vi "test_gmap-dot-net.vi"() -> ()   [LabVIEW 2019]
uses:
  C:/Users/WeGo/Documents/GitHub/Ycar/LabVIEW/Gmap/dll/GMap.NET.WindowsForms.dll
  dll/GMap.NET.WindowsForms.dll
  C:/Users/WeGo/Documents/GitHub/Ycar/LabVIEW/Gmap/dll/GMap.NET.Core.dll
  dll/GMap.NET.Core.dll
  System.Drawing
panel:
  in  "탭 컨트롤":enum32{"페이지 1", "페이지 2"}(tab)
  in  "SetMapProvider":u16(ring)=12 items=["None", "OpenStreetMap", "OpenStreet4UMap", "OpenCycleMap", "OpenCycleLandscapeMap", "OpenCycleTransportMap", "OpenStreetMapQuest", "OpenStreetMapQuestSattelite", "OpenStreetMapQuestHybrid", "OpenSeaMapHybrid", "WikiMapiaMap", "BingMap", "BingSatelliteMap", "BingHybridMap", "YahooMap", "YahooSatelliteMap", "YahooHybridMap", "GoogleMap", "GoogleSatelliteMap", "GoogleHybridMap", "GoogleTerrainMap", "GoogleChinaMap", "GoogleChinaSatelliteMap", "GoogleChinaHybridMap", "GoogleChinaTerrainMap", "GoogleKoreaMap", "GoogleKoreaSatelliteMap", "GoogleKoreaHybridMap", "NearMap", "NearSatelliteMap", "NearHybridMap", "OviMap", "OviSatelliteMap", "OviHybridMap", "OviTerrainMap", "YandexMap", "YandexSatelliteMap", "YandexHybridMap", "LithuaniaMap", "Lithuania 2.5d Map", "LithuaniaOrtoFotoMap", "LithuaniaOrtoFotoMapOld", "LithuaniaHybridMap", "LithuaniaHybridMapOld", "LithuaniaTOP50", "LatviaMap", "MapBender, WMS demo", "TurkeyMap", "CloudMade, Demo", "SpainMap", "CzechMap", "CzechSatelliteMap", "CzechHybridMap", "CzechTuristMap", "CzechHistoryMap", "ArcGIS_Imagery_World_2D_Map", "ArcGIS_ShadedRelief_World_2D_Map", "ArcGIS_StreetMap_World_2D_Map", "ArcGIS_Topo_US_2D_Map", "ArcGIS_World_Physical_Map", "ArcGIS_World_Shaded_Relief_Map", "ArcGIS_World_Street_Map", "ArcGIS_World_Terrain_Base_Map", "ArcGIS_World_Topo_Map", "ArcGIS_DarbAE_Q2_2011_NAVTQ_Eng_V5_MapProvider"]
  in  "GMapControl":refnum<k24>(container)
  in  "정지":bool
  in  "delay":u32=222
  in  "scale":dbl(slide) scale=0.0..20.0
  in  "keys":string
  out "SetPositionByKeywords":i32(ring)=200 items=["G_GEO_SUCCESS"=200, "G_GEO_BAD_REQUEST"=400, "G_GEO_SERVER_ERROR"=500, "G_GEO_MISSING_ADDRESS, G_GEO_MISSING_QUERY"=601, "G_GEO_UNKNOWN_ADDRESS"=602, "G_GEO_UNAVAILABLE_ADDRESS"=603, "G_GEO_UNKNOWN_DIRECTIONS"=604, "G_GEO_BAD_KEY"=610, "G_GEO_TOO_MANY_QUERIES"=620, "ExceptionInCode"=621, "Unknow"=-1]
  in  "MouseLat":dbl format="%.13f"
  in  "MouseLog":dbl format="%.13f"
  in  "MouseLat_DbClk":dbl format="%.13f"
  in  "MouseLog_DbClk":dbl format="%.13f"
  in  "PinDropLat_DblClk":dbl format="%.13f"
  in  "PinDropLon_DblClk":dbl format="%.13f"
  in  "dt":u32=150
  out "error out":errorcluster
  out "Contains":bool
  out "배열":cluster{string, string}[](array[cluster])
  out "Data":u8[](array[numeric])
  out "숫자형":i32
  out "Count":i32
  out "배열 2":T1(array[cluster])
  out "n":i32
  in  "keys 2":string
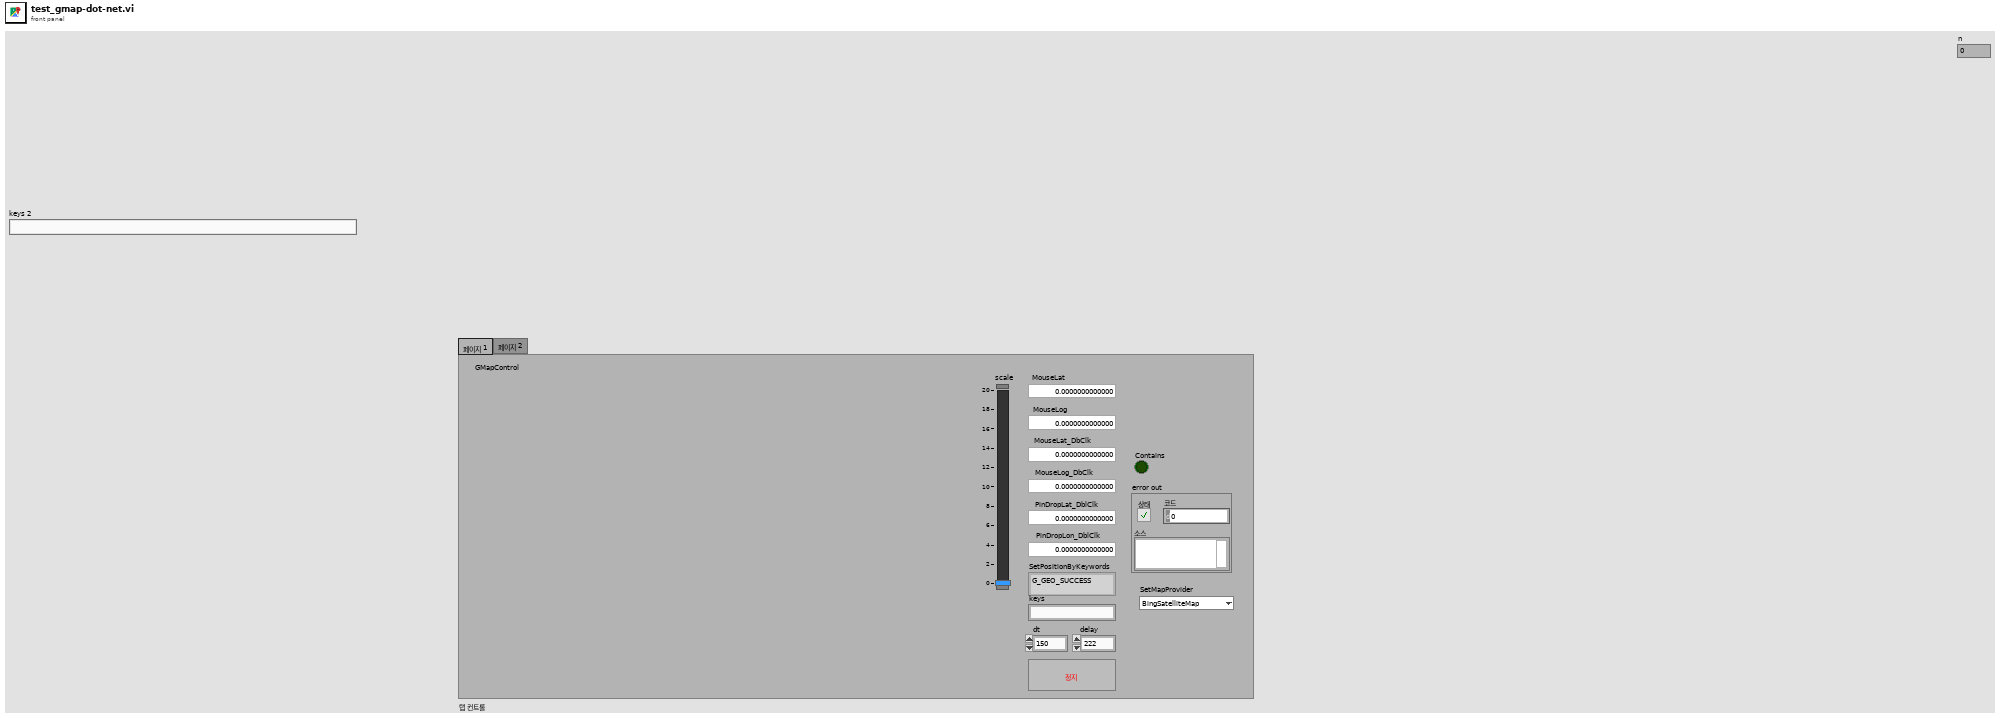
[diagram p1: front panel]
types:
  T1 = cluster{"index":i32, "dotnetrefs":refnum<k24>, "Name":string}[]
  T2 = typedef "mapinfo.ctl" = cluster{"GmapDotNet":refnum<k24>, "mapprovider_info":cluster{"index":i32, "dotnetrefs":refnum<k24>, "Name":string}[]}
  T3 = cluster{"index":i32, "dotnetrefs":refnum<k24>, "Name":string}
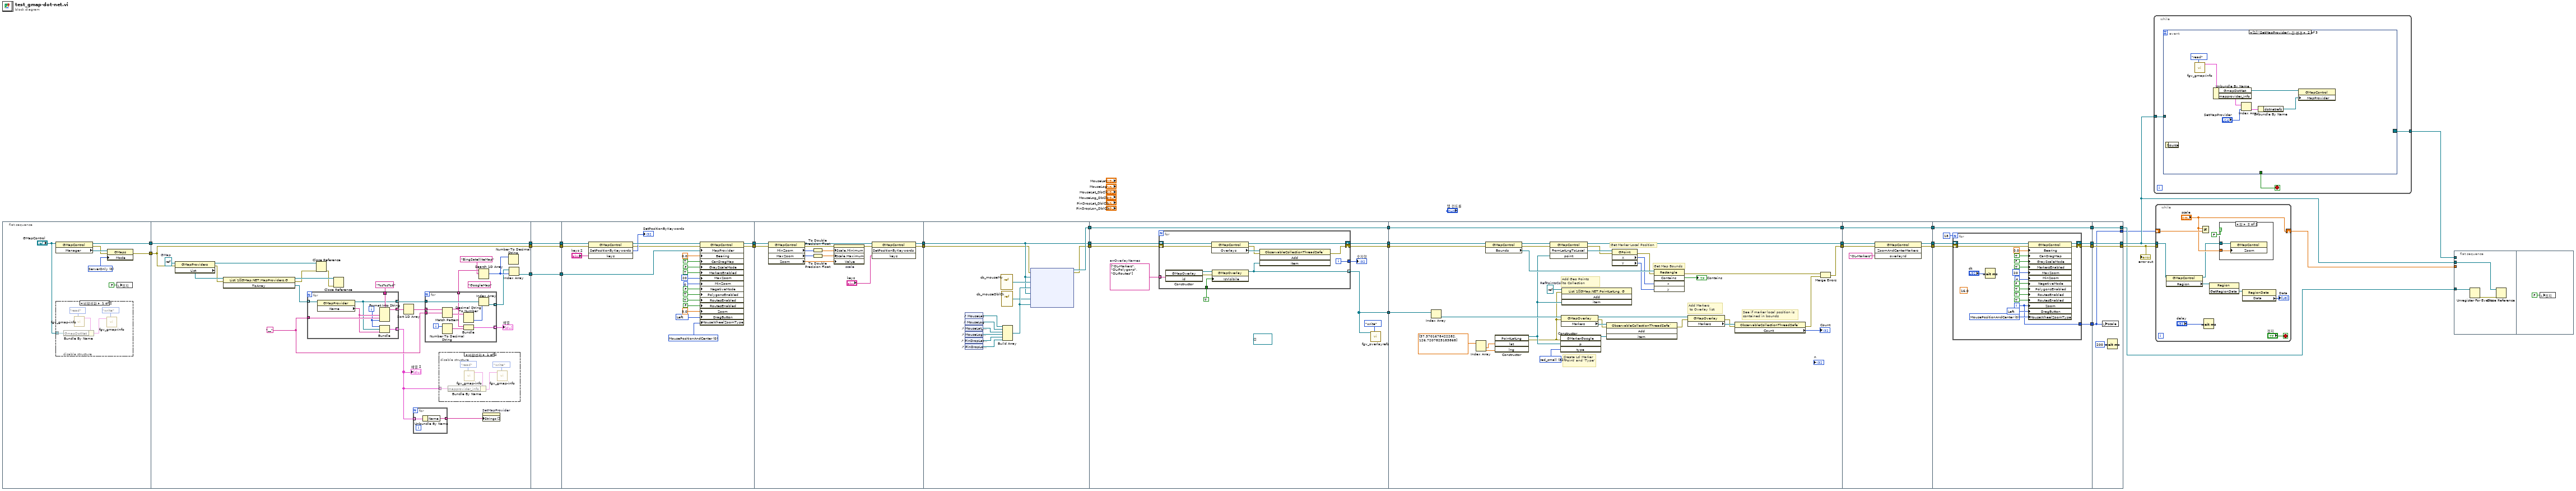
[diagram p0: block diagram]
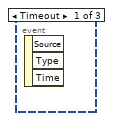
[diagram p2: hidden frame]
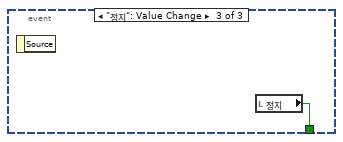
[diagram p3: hidden frame]
diagram:
  n1 = flat-sequence {
    tunnel: [w39] -> w35
    tunnel: [w38] -> w27
    tunnel: [w58] -> w33
    tunnel: w35 -> [w58]
    tunnel: [w57] -> w30
    tunnel: w27 -> [w50]
    tunnel: [w50] -> w26
    tunnel: w33 -> [w97]
    tunnel: [w97] -> w32
    tunnel: [w98] -> w31
    tunnel: w30 -> [w98]
    tunnel: w26 -> [w96]
    tunnel: [w96] -> w10
    tunnel: w32 -> [w101]
    tunnel: w31 -> [w104]
    tunnel: [w107] -> w29
    tunnel: [w106] -> w28
    tunnel: w10 -> [w100]
    tunnel: w29 -> [w127]
    tunnel: w28 -> [w128]
    tunnel: [w121] -> w25
    tunnel: [w123] -> w24
    tunnel: w25 -> [w135]
    tunnel: w24 -> [w136]
    tunnel: [w134] -> w21
    tunnel: [w136] -> w20
    tunnel: [w139] -> w19
    tunnel: w21 -> [w150]
    tunnel: w20 -> [w154]
    tunnel: w19 -> [w156]
    tunnel: [w149] -> w18
    tunnel: [w152] -> w17
    tunnel: [w156] -> w16
    tunnel: [w147] -> w14
    tunnel: w18 -> [w177]
    tunnel: w17 -> [w179]
    tunnel: w16 -> [w201]
    tunnel: w14 -> [w200]
    tunnel: [w170] -> w13
    tunnel: [w178] -> w12
    tunnel: [w201] -> w11
    tunnel: w13 -> [w203]
    tunnel: w12 -> [w205]
    tunnel: w11 -> [w207]
    tunnel: [w202] -> w9
    tunnel: [w204] -> w8
    tunnel: [w207] -> w7
    tunnel: w9 -> [w211]
    tunnel: w8 -> [w213]
    tunnel: w7 -> [w214]
    tunnel: [w210] -> w6
    tunnel: [w212] -> w5
    tunnel: [w214] -> w4
    tunnel: [w208] -> w3
    tunnel: [w235] -> w15
    tunnel: [w236] -> w22
    tunnel: [w237] -> w34
    tunnel: w6 -> [w237]
    tunnel: w5 -> [w236]
    tunnel: w4 -> [w235]
    tunnel: w3 -> [w233]
    tunnel: [w233] -> w2
    frame #0 {
      w40 = 0 items=["ServerOnly", "ServerAndCache", "CacheOnly"] ("Mode")
      n2 = property class="GMapControl"(reference="GMapControl") -> (reference out=w39:refnum<k24>, error out=w41:errorcluster, "Manager"=w42:refnum<k24>)  [unwired: 1 in]
      n3 = disable-structure shown="비활성화" {
        disable-tunnel: "GMapControl" -> [w44 _]
        frame Disabled {
          n4 = call "fgv_gmap-info.vi"("cmd"=enum16{"read", "write"}."read") -> ("mapinfo 2"=w45:T2)  [unwired: 9 in, 1 out]
          n5 = Bundle By Name(cluster=w45, "GmapDotNet"=w44) -> (w43:T2)
          n6 = call "fgv_gmap-info.vi"("cmd"=enum16{"read", "write"}."write", "mapinfo"=w43) -> ()  [unwired: 8 in, 2 out]
        }
        frame Enabled {
        }
      }
      n7 = property class="GMaps"(reference=w42, error in=w41, "Mode"=w40) -> (error out=w38:errorcluster)  [unwired: 1 out]
      n8 = local write "정지"(FALSE ("정지")) -> ()
    }
    frame #1 {
      (unwired) "GoogleMap" ("InitProviders")
      w65 = "__" ("regular expression")
      w60 = refnum<k24> refnum  # GMap
      n9 = property class="GMapProviders"(reference=w60, error in=w50) -> (reference out=w55:refnum<k24>, error out=w53:errorcluster, "List"=w69:refnum<k24>)
      n10 = invoke class="List`1[[GMap.NET.MapProviders.G" method="ToArray"(reference=w69, error in=w53) -> (reference out=w56:refnum<k24>, error out=w52:errorcluster, "ToArray"=w70:refnum<k24>[])  [unwired: 1 in]
      n11 = for {
        tunnel: w70 -> [w90] mode=indexing
        tunnel: [w95] -> w67 mode=indexing
        tunnel: [w88] -> w68 mode=indexing
        tunnel: "%s%s%d" ("format string") -> [w94]
        tunnel: w65 -> [w93]
        tunnel: [w89] -> w49 mode=indexing
        i -> [w91]
        n12 = property class="GMapProvider"(reference=w90) -> (reference out=w88:refnum<k24>, "Name"=w92:string)  [unwired: 1 in, 1 out]
        n13 = Format Into String(format string=w94, w92, w93, w91) -> (resulting string=w95:string)  [unwired: 2 in, 1 out]
        n14 = Bundle(w91, w88, "Name"=w92) -> (w89:cluster{i32, refnum<k24>, "Name":string})  [unwired: 1 in]
      }
      "배열 2" <- w49
      n15 = Close Reference(reference=w55, error in (no error)=w52) -> (error out=w51:errorcluster)
      n16 = Close Reference(reference=w56, error in (no error)=w51) -> ()  [unwired: 1 out]
      n17 = Sort 1D Array(array=w67) -> (sorted array=w64:string[])
      n18 = for {
        tunnel: w49 -> [w77] mode=indexing
        tunnel: [w76] -> w48 mode=indexing
        n19 = Unbundle By Name(w77) -> ("Name"=w76:string)
      }
      n20 = for {
        tunnel: w64 -> [w84] mode=indexing
        tunnel: [w85] -> w59 mode=indexing
        tunnel: w68 -> [w82]
        tunnel: [w80] -> w61 mode=indexing
        tunnel: w65 -> [w79]
        tunnel: [w78] -> w63 mode=indexing
        i -> [w86]
        n21 = Match Pattern(string=w84, regular expression=w79) -> (before substring=w78:string, after substring=w83:string)  [unwired: 1 in, 2 out]
        n22 = Number To Decimal String(number=w86) -> (decimal integer string=w87:string)  [unwired: 1 in]
        n23 = Bundle(w78, w87) -> (w85:cluster{string, string})  [unwired: 1 in]
        n24 = Decimal String To Number(string=w83) -> (number=w81:i32)  [unwired: 2 in, 1 out]
        n25 = Index Array(array=w82, index=w81) -> (element=w80:refnum<k24>)
      }
      "배열" <- w59
      n26 = disable-structure shown="비활성화" {
        disable-tunnel: w49 -> [w71 _]
        frame Disabled {
          n27 = call "fgv_gmap-info.vi"("cmd"=enum16{"read", "write"}."read") -> ("mapinfo 2"=w74:T2)  [unwired: 9 in, 1 out]
          n28 = Bundle By Name(cluster=w74, "mapprovider_info"=w71) -> (w72:T2)
          n29 = call "fgv_gmap-info.vi"("cmd"=enum16{"read", "write"}."write", "mapinfo"=w72) -> ()  [unwired: 8 in, 2 out]
        }
        frame Enabled {
        }
      }
      n30 = Search 1D Array(1D array=w63, element="BingSatelliteMap") -> (index of element=w62:i32)  [unwired: 1 in]
      n31 = property on="SetMapProvider" class="Ring (엄격한)"("Strings []"=w48) -> ()  [unwired: 2 in, 2 out]
      n32 = Number To Decimal String(number=w62) -> ()  [unwired: 1 in, 1 out]
      n33 = Index Array(array=w61, index=w62) -> (element=w57:refnum<k24>)
    }
    frame #2 {
    }
    frame #3 {
      w110 = 1048576 items=["None"=0, "Left"=1048576, "Right"=2097152, "Middle"=4194304, "XButton1"=8388608, "XButton2"=16777216] ("DragButton")
      w117 = 0 items=["MousePositionAndCenter", "MousePositionWithoutCenter", "ViewCenter"] ("MouseWheelZoomType")
      n34 = invoke class="GMapControl" method="SetPositionByKeywords"(reference=w101, error in=w100, "keys"="keys 2") -> (reference out=w103:refnum<k24>, error out=w99:errorcluster, "SetPositionByKeywords"=→"SetPositionByKeywords":i32)  [unwired: 1 in, 1 out]
      n35 = property class="GMapControl"(reference=w103, error in=w99, "MapProvider"=w104, "Bearing"=sgl 0.0, "CanDragMap"=TRUE, "GrayScaleMode"=FALSE ("CanDragMap"), "MarkersEnabled"=TRUE, "MaxZoom"=20, "MinZoom"=0, "NegativeMode"=FALSE, "PolygonsEnabled"=TRUE, "RoutesEnabled"=TRUE, "RoutesEnabled"=FALSE, "Zoom"=5.0, "DragButton"=w110, "MouseWheelZoomType"=w117) -> (reference out=w106:refnum<k24>, error out=w107:errorcluster)
    }
    frame #4 {
      n36 = property class="GMapControl"(reference=w128, error in=w127) -> (reference out=w125:refnum<k24>, error out=w126:errorcluster, "MinZoom"=w132:i32, "MaxZoom"=w131:i32, "Zoom"=w133:dbl)
      n37 = To Double Precision Float(number=w132) -> (double precision float=w130:dbl)
      n38 = To Double Precision Float(number=w131) -> (double precision float=w129:dbl)
      n39 = property on="scale" class="Slide (엄격한)"(error in=w126, "Scale.Minimum"=w130, "Scale.Maximum"=w129, "Value"=w133) -> (error out=w122:errorcluster)  [unwired: 1 in, 1 out]
      n40 = invoke class="GMapControl" method="SetPositionByKeywords"(reference=w125, error in=w122, "keys"="keys") -> (reference out=w123:refnum<k24>, error out=w121:errorcluster)  [unwired: 1 in, 2 out]
    }
    frame #5 {
      n41 = control-ref of="MouseLat"() -> (w145:refnum<vi>)
      n42 = control-ref of="MouseLog"() -> (w144:refnum<vi>)
      n43 = control-ref of="MouseLat_DbClk"() -> (w143:refnum<vi>)
      n44 = control-ref of="MouseLog_DbClk"() -> (w142:refnum<vi>)
      n45 = control-ref of="PinDropLat_DblClk"() -> (w146:refnum<vi>)
      n46 = control-ref of="PinDropLon_DblClk"() -> (w141:refnum<vi>)
      n47 = vi-ref "cb_mouseMv.vi"() -> ("vi reference"=w140:refnum<vi>)
      n48 = vi-ref "cb_mouseDblCk.vi"() -> ("vi reference"=w137:refnum<vi>)
      n49 = Build Array(w145, w144, w143, w142, w146, w141) -> (w138:refnum<vi>[])
      n50 = node(w135, w136, w140, w138, w136, w137, w138) -> (w139:refnum<k27>, w134:errorcluster)  [unwired: 1 in]
    }
    frame #6 {
      (unwired) refnum<k24>[] []
      w153 = string[] ["OL-Markers", "OL-Polygons", "OL-Routes"]  # arrOverlayNames
      n51 = for {
        tunnel: w153 -> [w168] mode=indexing
        tunnel: [w162] -> w147 mode=indexing
        shift-right: [w165] -> w152
        shift-left: w154 -> [w167]
        tunnel: TRUE ("IsVisibile") -> [w164]
        tunnel: [w161] -> w151
        shift-right: [w158] -> w149
        shift-left: w150 -> [w160]
        i -> [w161]
        n52 = constructor class="GMapOverlay"("id"=w168) -> (reference out=w163:refnum<k24>, error out=w157:errorcluster)  [unwired: 3 in, 2 out]
        n53 = property class="GMapControl"(reference=w167, error in=w160) -> (reference out=w165:refnum<k24>, error out=w159:errorcluster, "Overlays"=w166:refnum<k24>)
        n54 = property class="GMapOverlay"(reference=w163, error in=w157, "IsVisibile"=w164) -> (reference out=w162:refnum<k24>)  [unwired: 1 out]
        n55 = invoke class="ObservableCollectionThreadSafe`" method="Add"(reference=w166, error in=w159, "item"=w162) -> (error out=w158:errorcluster)  [unwired: 1 in, 3 out]
      }
      "숫자형" <- w151
      n56 = call "fgv_overlayrefs.vi"("cmd"=enum16{"read", "write"}."write", "overlayrefs"=w147) -> ()  [unwired: 9 in, 1 out]
    }
    frame #7 {
      w199 = 32 items=["none", "arrow", "blue", "blue_small", "blue_dot", "blue_pushpin", "brown_small", "gray_small", "green", "green_small", "green_dot", "green_pushpin", "green_big_go", "yellow", "yellow_small", "yellow_dot", "yellow_big_pause", "yellow_pushpin", "lightblue", "lightblue_dot", "lightblue_pushpin", "orange", "orange_small", "orange_dot", "pink", "pink_dot", "pink_pushpin", "purple", "purple_small", "purple_dot", "purple_pushpin", "red", "red_small", "red_dot", "red_pushpin", "red_big_stop", "black_small", "white_small"] ("type")
      w197 = refnum<k24> refnum  # RefPointsColl
      # "See if marker local position is \ncontained in bounds"
      # "Get Marker Local Position"
      # "Get Map Bounds"
      # "Add Markers\n to Overlay list"
      # "Create Lcl Marker  'Point' and 'Type'"
      # "Add Geo Points\n to Collection"
      n57 = Index Array(array=w200) -> (element=w198:refnum<k24>)  [unwired: 1 in]
      n58 = Index Array(array=dbl[] [37.3701678422282, 126.7207825183868] ("arrLatLngActv")) -> (element #1=w185:dbl, element #2=w184:dbl)  [unwired: 2 in]
      n59 = property class="GMapControl"(reference=w179, error in=w177) -> (reference out=w187:refnum<k24>, error out=w183:errorcluster, "Bounds"=w192:refnum<k24>)
      n60 = constructor class="PointLatLng"("lat"=w185, "lng"=w184) -> (reference out=w176:refnum<k24>, error out=w169:errorcluster)  [unwired: 3 in, 3 out]
      n61 = invoke class="GMapControl" method="FromLatLngToLocal"(reference=w187, error in=w183, "point"=w176) -> (reference out=w178:refnum<k24>, error out=w182:errorcluster, "FromLatLngToLocal"=w190:refnum<k24>)  [unwired: 1 in, 1 out]
      n62 = constructor class="GMarkerGoogle"(error in=w169, "p"=w176, "type"=w199) -> (reference out=w191:refnum<k24>)  [unwired: 2 in, 4 out]
      n63 = property class="GMapOverlay"(reference=w198, error in=w169) -> (reference out=w195:refnum<k24>, error out=w175:errorcluster, "Markers"=w193:refnum<k24>)
      n64 = invoke class="List`1[[GMap.NET.PointLatLng, G" method="Add"(reference=w197, error in=w169, "item"=w176) -> ()  [unwired: 1 in, 4 out]
      n65 = invoke class="ObservableCollectionThreadSafe`" method="Add"(reference=w193, error in=w175, "item"=w191) -> (error out=w174:errorcluster)  [unwired: 1 in, 3 out]
      n66 = property class="GPoint"(reference=w190, error in=w182) -> (error out=w181:errorcluster, "X"=w189:i64, "Y"=w188:i64)  [unwired: 1 out]
      n67 = invoke class="Rectangle" method="Contains"(reference=w192, error in=w181, "x"=w189, "y"=w188) -> (error out=w172:errorcluster, "Contains"=→"Contains":bool)  [unwired: 1 in, 3 out]
      n68 = property class="GMapOverlay"(reference=w195, error in=w174) -> (error out=w173:errorcluster, "Markers"=w196:refnum<k24>)  [unwired: 1 out]
      n69 = property class="ObservableCollectionThreadSafe`"(reference=w196, error in=w173) -> (error out=w171:errorcluster, "Count"=→"Count":i32)  [unwired: 1 out]
      n70 = Merge Errors(w172, w171) -> (w170:errorcluster)
    }
    frame #8 {
      n71 = invoke class="GMapControl" method="ZoomAndCenterMarkers"(reference=w205, error in=w203, "overlayId"="OL-Markers") -> (reference out=w204:refnum<k24>, error out=w202:errorcluster)  [unwired: 1 in, 2 out]
    }
    frame #9 {
      n72 = for {
        N: 18 -> [_]
        shift-right: [w219] -> w212
        shift-left: w213 -> [w220]
        shift-right: [w217] -> w210
        shift-left: w211 -> [w218]
        tunnel: [w215] -> w208
        i -> [w215]
        w221 = 1048576 items=["None"=0, "Left"=1048576, "Right"=2097152, "Middle"=4194304, "XButton1"=8388608, "XButton2"=16777216] ("DragButton")
        (unwired) 16.0 ("Zoom")
        w227 = 0 items=["MousePositionAndCenter", "MousePositionWithoutCenter", "ViewCenter"] ("MouseWheelZoomType")
        n73 = Wait (ms)(milliseconds to wait="dt") -> ()  [unwired: 1 out]
        n74 = property class="GMapControl"(reference=w220, error in=w218, "Bearing"=sgl 0.0, "CanDragMap"=TRUE, "GrayScaleMode"=FALSE ("CanDragMap"), "MarkersEnabled"=TRUE, "MaxZoom"=20, "MinZoom"=4, "NegativeMode"=FALSE, "PolygonsEnabled"=TRUE, "RoutesEnabled"=TRUE, "RoutesEnabled"=TRUE, "Zoom"=w215, "DragButton"=w221, "MouseWheelZoomType"=w227) -> (reference out=w219:refnum<k24>, error out=w217:errorcluster)
      }
    }
    frame #10 {
      n75 = local write "scale"(w233) -> ()
      n76 = Wait (ms)(milliseconds to wait=u32 200 ("대기 시간 (ms)")) -> ()  [unwired: 1 out]
    }
  }
  n77 = while {
    tunnel: w22 -> [w239]
    tunnel: [w238] -> w1
    stop <- w240 stop-if-true
    n78 = event shown="[1] \"SetMapProvider\": 값 변경" {
      selector: _ -> [_ _ _]
      dyn-events: [_ _ _] -> w238
      timeout: _ -> [_ _ _]
      tunnel: [_ _ w248] -> w240
      tunnel: w239 -> [_ _ _]
      event Timeout {
        n79 = event-data() -> ()  [unwired: 1 in, 3 out]
      }
      event "SetMapProvider": Value Change {
        n80 = event-data() -> ()  [unwired: 1 in, 1 out]
        n81 = call "fgv_gmap-info.vi"("cmd"=enum16{"read", "write"}."read") -> ("mapinfo 2"=w243:T2)  [unwired: 9 in, 1 out]
        n82 = Unbundle By Name(w243) -> ("GmapDotNet"=w242:refnum<k24>, "mapprovider_info"=w246:T1)
        n83 = Index Array(array=w246, index="SetMapProvider") -> (element=w244:T3)
        n84 = Unbundle By Name(w244) -> ("dotnetrefs"=w241:refnum<k24>)
        n85 = property class="GMapControl"(reference=w242, "MapProvider"=w241) -> ()  [unwired: 1 in, 2 out]
      }
      event "정지": Value Change {
        n86 = event-data() -> ()  [unwired: 1 in, 1 out]
        n87 = local read "정지"() -> (w248:bool)
      }
    }
  }
  n88 = while {
    tunnel: w34 -> [_]
    tunnel: w22 -> [w254]
    shift-right: ["scale"] -> w23
    shift-left: w2 -> [w256]
    stop <- "정지" stop-if-true
    n89 = property class="GMapControl"(reference=w254) -> (reference out=w249:refnum<k24>, "Region"=w253:refnum<k24>)  [unwired: 1 in, 1 out]
    n90 = Not Equal?(x="scale", y=w256) -> ()  [unwired: 1 out]
    n91 = Wait (ms)(milliseconds to wait="delay") -> ()  [unwired: 1 out]
    n92 = invoke class="Region" method="GetRegionData"(reference=w253) -> ("GetRegionData"=w252:refnum<k24>)  [unwired: 2 in, 2 out]
    n93 = case shown="참" FALSE {
      tunnel: w249 -> [_ w260]
      tunnel: "scale" -> [_ w259]
      frame False {
      }
      frame True {
        n94 = property class="GMapControl"(reference=w260, "Zoom"=w259) -> ()  [unwired: 1 in, 2 out]
      }
    }
    n95 = property class="RegionData"(reference=w252) -> ("Data"=→"Data":u8[])  [unwired: 1 in, 2 out]
  }
  n96 = flat-sequence {
    tunnel: w15 -> [w263]
    tunnel: w23 -> [_]
    tunnel: w22 -> [w261]
    tunnel: w1 -> [_]
    frame #0 {
      n97 = Unregister For Events(event registration refnum=w263) -> (error out=w262:errorcluster)  [unwired: 1 in]
      n98 = Close Reference(reference=w261, error in (no error)=w262) -> ()  [unwired: 1 out]
    }
    frame #1 {
      n99 = local write "정지"(FALSE ("정지")) -> ()
    }
  }
  "error out" <- w34
